vi "izmeri_zapreminu.vi"(0 "task in":refnum<k21>, 11 "error in":errorcluster) -> (4 "task out":refnum<k21>, 6 "trajanje[s]":dbl, 8 "V":dbl, 10 "prekinut":bool=TRUE, 15 "error out":errorcluster)   [LabVIEW 2019]
doc: "Merenje dostupne količine vode pomoću senzora sile. \nNapon koji se meri je u opsegu od 0 do 5V, tako da je količina vode u opsegu od 0 do približno 600ml. Korisnik bira vrstu kafe - za kraći espresso potrebno je 40ml, za duži 110ml. Ako se izmeri manje vraća se greška.\nUlaz: port uređaja koji se koristi kao senzor sile.\nIzlazi: izmerena količina vode, prekinuta operacija i greška."
uses:
  <vilib>/DAQmx/read.llb/DAQmx Read (Analog DBL 1Chan 1Samp).vi
  <vilib>/DAQmx/miscellaneous.llb/DAQmx Fill In Error Info.vi
panel:
  in  "duzi":bool
  in  "kraci":bool
  # "Izaberite željenu kafu:"
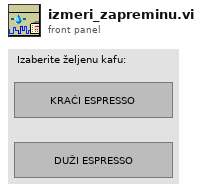
[diagram p1: front panel]
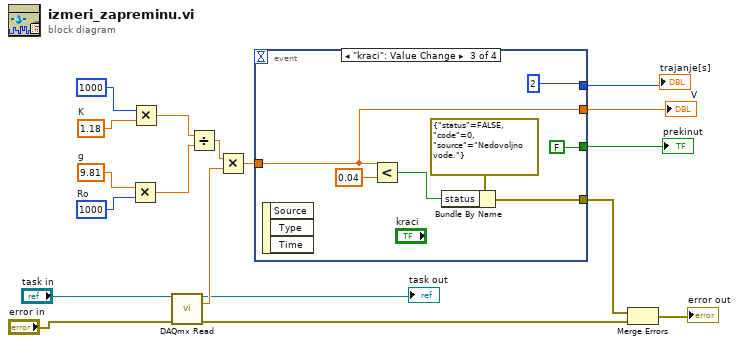
[diagram p0: block diagram]
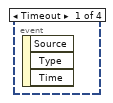
[diagram p2: hidden frame]
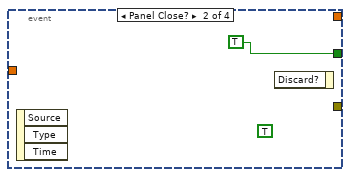
[diagram p3: hidden frame]
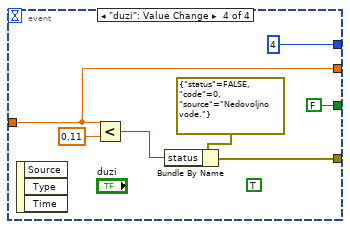
[diagram p4: hidden frame]
diagram:
  w9 = 1000  # Ro
  w8 = 9.81  # g
  w7 = 1.18  # K
  n1 = Multiply(x=w8, y=w9) -> (x*y=w10:dbl)
  n2 = Multiply(x=1000, y=w7) -> (x*y=w11:dbl)
  n3 = call-poly <vilib>:"DAQmx Read.vi"("task/channels in"="task in", "error in"="error in") -> ("task out"=→"task out":refnum<k21>, "data"=w13:dbl, "error out"=w3:errorcluster)  [unwired: 11 in]
  n4 = Divide(x=w11, y=w10) -> (x/y=w5:dbl)
  n5 = Multiply(x=w5, y=w13) -> (x*y=w12:dbl)
  n6 = event shown="[2] \"kraci\": Value Change" {
    selector: _ -> [_ _ _ _]
    dyn-events: _ -> [_ _ _ _]
    timeout: _ -> [_ _ _ _]
    tunnel: w12 -> [_ _ w25 w30]
    tunnel: [_ _ w25 w30] -> w18
    tunnel: [_ _ w22 w29] -> w2
    tunnel: [_ TRUE FALSE FALSE] -> w17
    tunnel: [_ _ 2 4] -> w16
    event Timeout {
      n7 = event-data() -> ()  [unwired: 1 in, 3 out]
    }
    event Panel Close? {
      (unwired) TRUE
      n8 = event-data() -> ()  [unwired: 1 in, 3 out]
      n9 = event-data() -> ()  [unwired: 2 in, 1 out]
    }
    event "kraci": Value Change {
      n10 = event-data() -> ()  [unwired: 1 in, 3 out]
      n11 = Less?(x=w25, y=0.04) -> (x < y?=w24:bool)
      n12 = Bundle By Name(cluster=errorcluster {"status"=FALSE, "code"=0, "source"="Nedovoljno vode."} ("error constant"), "status"=w24) -> (w22:errorcluster)
    }
    event "duzi": Value Change {
      (unwired) TRUE
      n13 = event-data() -> ()  [unwired: 1 in, 3 out]
      n14 = Less?(x=w30, y=0.11) -> (x < y?=w32:bool)
      n15 = Bundle By Name(cluster=errorcluster {"status"=FALSE, "code"=0, "source"="Nedovoljno vode."} ("error constant"), "status"=w32) -> (w29:errorcluster)
    }
  }
  "V" <- w18
  "prekinut" <- w17
  "trajanje[s]" <- w16
  n16 = Merge Errors(w2, w3) -> (→"error out":errorcluster)
